vi "openKuka.vi"(10 "远程端口或服务名称":u16, 11 "地址":string) -> (0 "错误输出":errorcluster, 3 "TCP网络连接输出":refnum<k5>)   [LabVIEW 2015, in "labOpenShowVar.lvlib"]
doc: "打开tcp连接"
uses:
  labOpenShowVar.lvlib
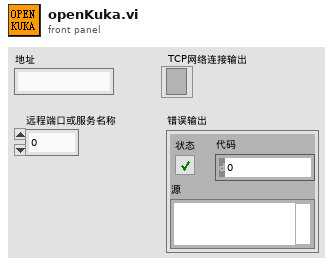
[diagram p1: front panel]
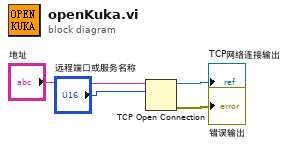
[diagram p0: block diagram]
diagram:
  n1 = TCP Open Connection(address="地址", remote port or service name="远程端口或服务名称") -> (connection ID=→"TCP网络连接输出":refnum<k5>, error out=→"错误输出":errorcluster)  [unwired: 3 in]
